vi "testMinMax.vi"(8 "error in (no error)":errorcluster, 10 "passThreshold":i32[](array[numeric]), 11 "reference in":refnum<class "subject.lvclass">) -> (0 "error out":errorcluster, 3 "reference out":refnum<class "subject.lvclass">)   [LabVIEW 2015, in "subject.lvclass"]
uses:
  subject.lvclass
panel:
  in  "valesAmplitude in":dbl[](array[numeric])
  in  "peaksAmplitude in":dbl[](array[numeric])
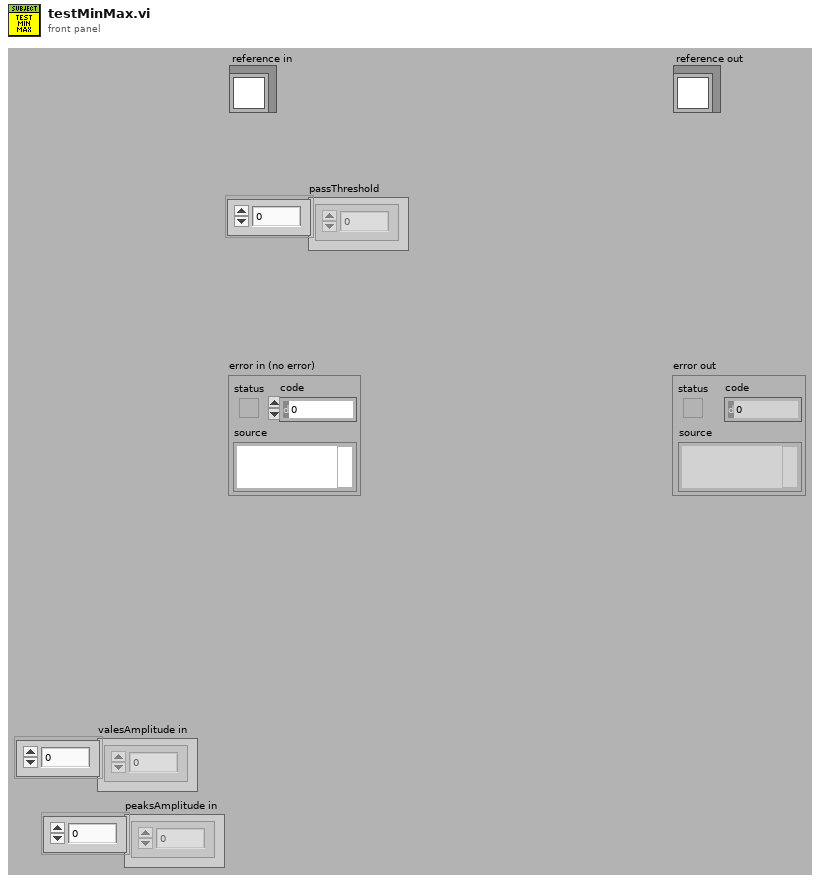
[diagram p1: front panel]
types:
  T1 = cluster{"peaksAmplitude":dbl[], "iPeaksLocation":dbl[], "valesAmplitude":dbl[], "iValesLocation":dbl[], "threshold":dbl, "width_warm":i32, "meanAmpl_warm":i32, "#_peaks":i32}
  T2 = typedef "subject.lvclass/ObjectAttributesRef.ctl" = refnum<data-value>
  T3 = typedef "subject.lvclass/ObjectAttributes.ctl" = cluster{"MyAttribute":dbl, "data":cluster{"Ve_warm":dbl[], "time_warm":dbl[], "name":string, "phase":dbl[], "VCO2":dbl[], "VO2":dbl[], "PetCO2":dbl[], "RQ":dbl[], "HR":dbl[], "Ve_warm_inter":dbl[], "time_warm_inter":dbl[], "Ve_exer":dbl[], "time_exer":dbl[], "Ve_exer_inter":dbl[], "time_exer_inter":dbl[], "Ve":dbl[], "time":dbl[]}, "results_5l":cluster{"EOV":bool, "osci_amplitude":dbl[], "osci_width":dbl[], "peak_location":dbl[], "threshold":dbl, "width":i32}, "results_15percent":cluster{"EOV":bool, "osci_amplitude":dbl[], "osci_width":dbl[], "peak_location":dbl[], "threshold":dbl, "width":i32}, "supportData":cluster{"peaksAmplitude":dbl[], "iPeaksLocation":dbl[], "valesAmplitude":dbl[], "iValesLocation":dbl[], "threshold":dbl, "meanAmpl_warm":i32, "#_peaks":i32, "width":i32}, "results_user_selection":cluster{"EOV":bool, "osci_amplitude":dbl[], "osci_width":dbl[], "peak_location":dbl[], "threshold":dbl, "width":i32}}
  T4 = cluster{"peaksAmplitude":dbl[], "iPeaksLocation":dbl[], "valesAmplitude":dbl[], "iValesLocation":dbl[], "threshold":dbl, "meanAmpl_warm":i32, "#_peaks":i32, "width":i32}
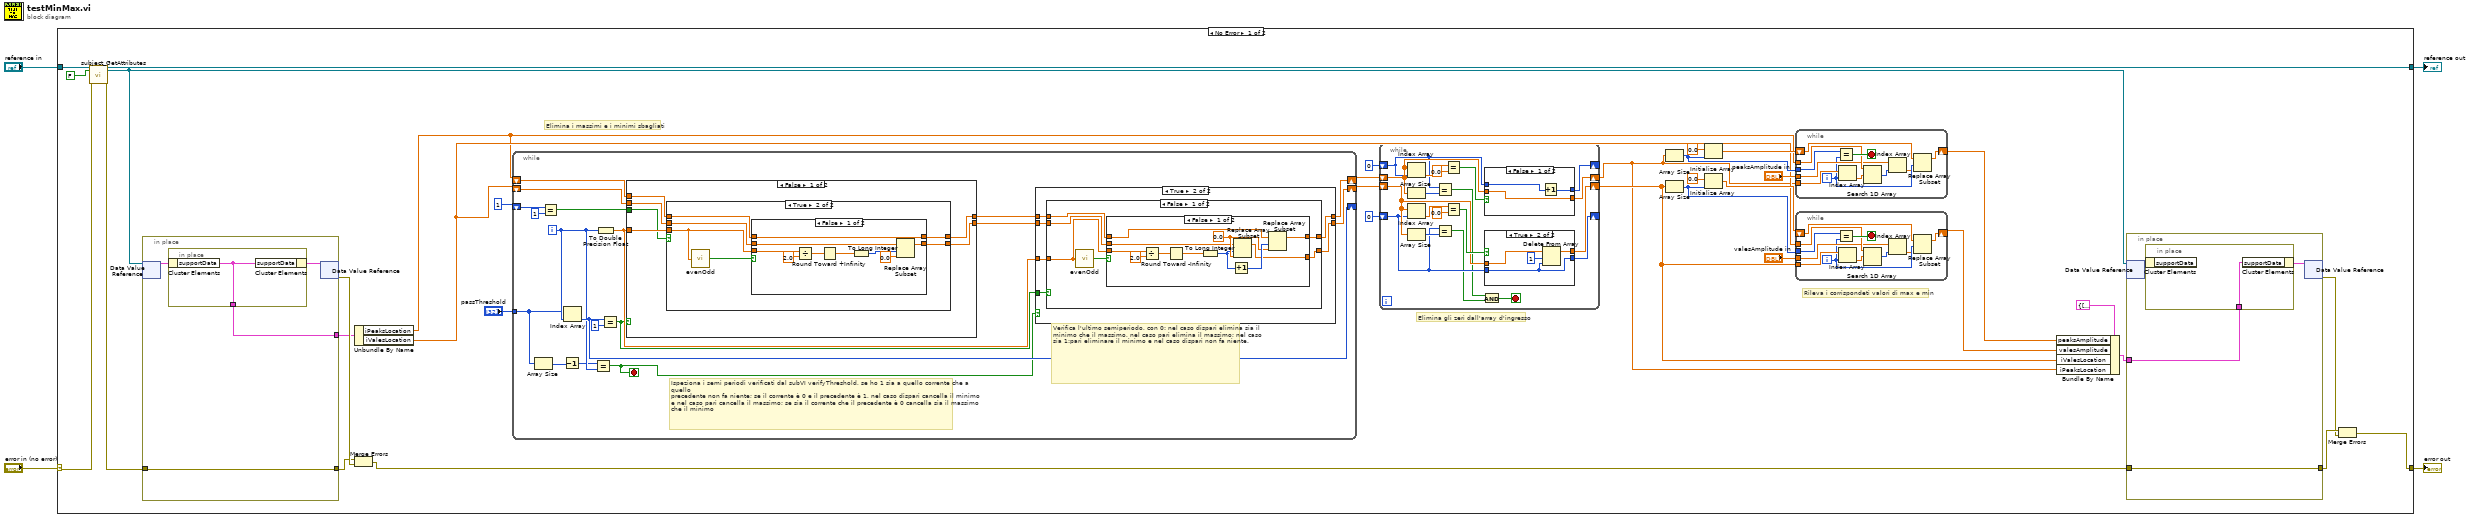
[diagram p0: block diagram]
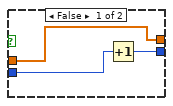
[diagram p2: hidden frame]
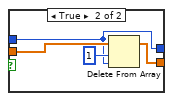
[diagram p3: hidden frame]
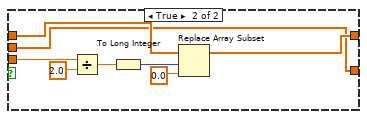
[diagram p5: hidden frame]
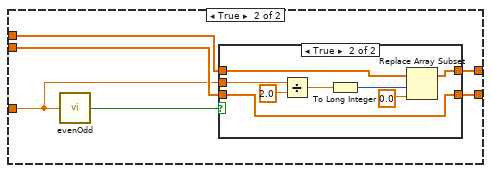
[diagram p6: hidden frame]
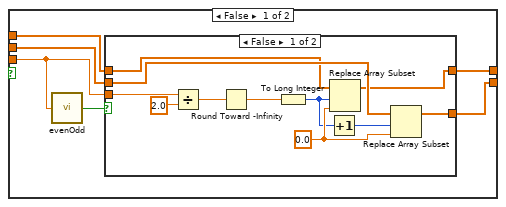
[diagram p8: hidden frame]
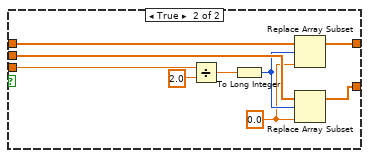
[diagram p9: hidden frame]
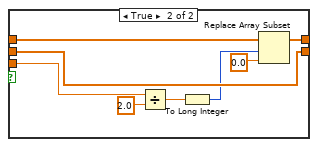
[diagram p10: hidden frame]
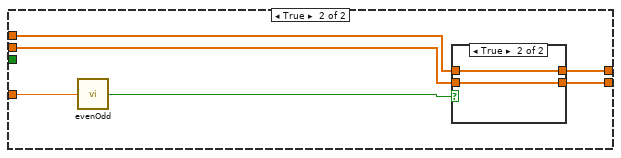
[diagram p11: hidden frame]
diagram:
  n1 = case shown="No Error" "error in (no error)" {
    selector: "error in (no error)" -> [w35 w238]
    tunnel: [w12 w238] -> w3
    tunnel: [w33 w237] -> w1
    tunnel: "reference in" -> [w37 w237]
    frame No Error {
      # "Rileva i corrispondeti valori di max e min"
      # "Elimina gli zeri dall'array d'ingresso"
      # "Elimina i massimi e i minimi sbagliati"
      n2 = call "subject_GetAttributes.vi"("reference in"=w37, "return data? (T)"=FALSE, "error in (no error)"=w35) -> ("reference out"=w33:refnum<class "subject.lvclass">, "attributes ref"=w11:T2, "error out"=w34:errorcluster)  [unwired: 13 in, 1 out]
      n3 = in-place {
        in-place-border: w34 -> [w233]
        in-place-border: [w233] -> w38
        in-place-border: [w232] -> w18
        n4 = in-place-dvr #1(w11) -> (w234:T3)  [unwired: 1 out]
        n5 = in-place {
          in-place-border: [w236] -> w232
          n6 = in-place-cluster #2(w234) -> ("supportData"=w236:T4)
          n7 = in-place-cluster #2("supportData"=w236) -> (w235:T3)
        }
        n8 = in-place-dvr #1(w235) -> (w39:errorcluster)  [unwired: 1 out]
      }
      n9 = Unbundle By Name(w18) -> ("iPeaksLocation"=w16:dbl[], "iValesLocation"=w17:dbl[])
      n10 = Merge Errors(w38, w39) -> (w15:errorcluster)
      n11 = while {
        tunnel: "passThreshold" -> [w101]
        shift-right: [w104] -> w29
        shift-left: w16 -> [w116]
        shift-right: [w105] -> w30
        shift-left: w17 -> [w115]
        shift-right: [w114] -> _
        shift-left: 1 ("element") -> [w113]
        i -> [w110]
        stop <- w106 stop-if-true
        # "Verifica l'ultimo semiperiodo, con 0: nel caso dispari elimina sia il minimo che il massimo, nel caso pari elimina il massimo; nel caso sia 1:pari eliminare il minimo e nel caso dispari non fa niente."
        # "Ispeziona i semi periodi verificati dal subVI verifyThreshold, se ho 1 sia a quello corrente che a quello \nprecedente non fa niente; se il corrente è 0 e il precedente è 1, nel caso dispari cancella il minimo e nel caso pari cancella il massimo; se sia il corrente che il precedente è 0 cancella sia il massimo che il minimo"
        n12 = Array Size(array=w101) -> (size(s)=w109:i32)
        n13 = Equal?(x=w113, y=1) -> (x = y?=w111:bool)
        n14 = Decrement(x=w109) -> (x-1=w103:i32)
        n15 = Index Array(array=w101, index=w110) -> (element=w114:i32)
        n16 = Equal?(x=w103, y=w110) -> (x = y?=w106:bool)
        n17 = To Double Precision Float(number=w110) -> (double precision float=w102:dbl)
        n18 = Equal?(x=w114, y=1) -> (x = y?=w100:bool)
        n19 = case shown="False" w100 {
          tunnel: w102 -> [w172 w227]
          tunnel: w116 -> [w171 w225]
          tunnel: w115 -> [w170 w223]
          tunnel: [w169 w224] -> w107
          tunnel: [w168 w222] -> w108
          tunnel: w111 -> [w167 _]
          frame False {
            n20 = case shown="True" w167 {
              tunnel: w172 -> [w173 w199]
              tunnel: w171 -> [w176 w203]
              tunnel: w170 -> [w178 w200]
              tunnel: [w175 w202] -> w169
              tunnel: [w177 w201] -> w168
              frame False {
                n21 = call "evenOdd.vi"("number"=w173) -> ("odd/even"=w174:bool)
                n22 = case shown="False" w174 {
                  tunnel: w178 -> [w189 w198]
                  tunnel: [w188 w197] -> w177
                  tunnel: w176 -> [w179 w196]
                  tunnel: [w187 w195] -> w175
                  tunnel: w173 -> [w186 w194]
                  frame False {
                    w182 = 0.0 ("new element/subarray")
                    n23 = Divide(x=w186, y=2.0) -> (x/y=w184:dbl)
                    n24 = Round Toward -Infinity(1:w184) -> (0:w183:dbl)
                    n25 = To Long Integer(number=w183) -> (32bit integer=w181:i32)
                    n26 = Increment(x=w181) -> (x+1=w180:i32)
                    n27 = Replace Array Subset(array=w179, new element=w182, index=w181) -> (w187:dbl[])
                    n28 = Replace Array Subset(array=w189, new element=w182, index=w180) -> (w188:dbl[])
                  }
                  frame True {
                    w190 = 0.0 ("new element/subarray")
                    n29 = Divide(x=w194, y=2.0) -> (x/y=w192:dbl)
                    n30 = To Long Integer(number=w192) -> (32bit integer=w191:i32)
                    n31 = Replace Array Subset(array=w196, new element=w190, index=w191) -> (w195:dbl[])
                    n32 = Replace Array Subset(array=w198, new element=w190, index=w191) -> (w197:dbl[])
                  }
                }
              }
              frame True {
                n33 = call "evenOdd.vi"("number"=w199) -> ("odd/even"=w204:bool)
                n34 = case shown="False" w204 {
                  tunnel: w203 -> [w211 w221]
                  tunnel: w200 -> [w213 w219]
                  tunnel: w199 -> [w209 w216]
                  tunnel: [w211 w220] -> w202
                  tunnel: [w212 w219] -> w201
                  frame False {
                    n35 = Divide(x=w209, y=2.0) -> (x/y=w207:dbl)
                    n36 = Round Toward +Infinity(x=w207) -> (ceil(x): smallest int >= x=w206:dbl)
                    n37 = To Long Integer(number=w206) -> (32bit integer=w205:i32)
                    n38 = Replace Array Subset(array=w213, new element=0.0 ("new element/subarray"), index=w205) -> (w212:dbl[])
                  }
                  frame True {
                    n39 = Divide(x=w216, y=2.0) -> (x/y=w214:dbl)
                    n40 = To Long Integer(number=w214) -> (32bit integer=w217:i32)
                    n41 = Replace Array Subset(array=w221, new element=0.0 ("length"), index=w217) -> (w220:dbl[])
                  }
                }
              }
            }
          }
          frame True {
            n42 = call "evenOdd.vi"("number"=w227) -> ("odd/even"=w226:bool)
            n43 = case shown="True" w226 {
              tunnel: w225 -> [w229 w231]
              tunnel: [w229 w231] -> w224
              tunnel: w223 -> [w228 w230]
              tunnel: [w228 w230] -> w222
              frame False {
              }
              frame True {
              }
            }
          }
        }
        n44 = case shown="True" w106 {
          tunnel: w108 -> [w119 w125]
          tunnel: w107 -> [w118 w122]
          tunnel: w102 -> [_ w124]
          tunnel: [w119 w123] -> w105
          tunnel: [w118 w121] -> w104
          tunnel: w100 -> [_ w120]
          frame False {
          }
          frame True {
            n45 = case shown="False" w120 {
              tunnel: w125 -> [w130 w155]
              tunnel: w124 -> [w126 w154]
              tunnel: [w128 w153] -> w123
              tunnel: w122 -> [w129 w152]
              tunnel: [w127 w151] -> w121
              frame False {
                n46 = call "evenOdd.vi"("number"=w126) -> ("odd/even"=w131:bool)
                n47 = case shown="False" w131 {
                  tunnel: w130 -> [w136 w148]
                  tunnel: w129 -> [w135 w150]
                  tunnel: [w134 w148] -> w128
                  tunnel: [w133 w149] -> w127
                  tunnel: w126 -> [w132 w147]
                  frame False {
                    w141 = 0.0 ("new element/subarray")
                    n48 = Divide(x=w132, y=2.0) -> (x/y=w138:dbl)
                    n49 = Round Toward -Infinity(1:w138) -> (0:w139:dbl)
                    n50 = To Long Integer(number=w139) -> (32bit integer=w140:i32)
                    n51 = Increment(x=w140) -> (x+1=w142:i32)
                    n52 = Replace Array Subset(array=w136, new element=w141, index=w140) -> (w134:dbl[])
                    n53 = Replace Array Subset(array=w135, new element=w141, index=w142) -> (w133:dbl[])
                  }
                  frame True {
                    n54 = Divide(x=w147, y=2.0) -> (x/y=w145:dbl)
                    n55 = To Long Integer(number=w145) -> (32bit integer=w144:i32)
                    n56 = Replace Array Subset(array=w150, new element=0.0 ("new element/subarray"), index=w144) -> (w149:dbl[])
                  }
                }
              }
              frame True {
                n57 = call "evenOdd.vi"("number"=w154) -> ("odd/even"=w156:bool)
                n58 = case shown="True" w156 {
                  tunnel: w155 -> [w157 w159]
                  tunnel: w154 -> [_ w166]
                  tunnel: [w157 w159] -> w153
                  tunnel: w152 -> [w158 w161]
                  tunnel: [w158 w160] -> w151
                  frame False {
                  }
                  frame True {
                    n59 = Divide(x=w166, y=2.0) -> (x/y=w164:dbl)
                    n60 = To Long Integer(number=w164) -> (32bit integer=w163:i32)
                    n61 = Replace Array Subset(array=w161, new element=0.0 ("new element/subarray"), index=w163) -> (w160:dbl[])
                  }
                }
              }
            }
          }
        }
      }
      n62 = while {
        shift-right: [w78] -> w7
        shift-left: w29 -> [w71]
        shift-right: [w79] -> w8
        shift-left: w30 -> [w75]
        shift-right: [w77] -> _
        shift-left: 0 -> [w73]
        shift-right: [w76] -> _
        shift-left: 0 -> [w67]
        stop <- w68 stop-if-true
        n63 = Index Array(array=w71, index=w67) -> (element=w85:dbl)
        n64 = Array Size(array=w71) -> (size(s)=w72:i32)
        n65 = Index Array(array=w75, index=w73) -> (element=w82:dbl)
        n66 = Array Size(array=w75) -> (size(s)=w74:i32)
        n67 = Equal?(x=w67, y=w72) -> (x = y?=w69:bool)
        n68 = Equal?(x=w73, y=w74) -> (x = y?=w70:bool)
        n69 = Equal?(x=w85, y=0.0) -> (x = y?=w83:bool)
        n70 = Equal?(x=w82, y=0.0) -> (x = y?=w80:bool)
        n71 = And(x=w69, y=w70) -> (x .and. y?=w68:bool)
        n72 = case shown="False" w83 {
          tunnel: w71 -> [w93 w99]
          tunnel: [w93 w98] -> w78
          tunnel: [w95 w96] -> w76
          tunnel: w67 -> [w94 w96]
          frame False {
            n73 = Increment(x=w94) -> (x+1=w95:i32)
          }
          frame True {
            n74 = Delete From Array(array=w99, length=1, index=w96) -> (array with subset deleted=w98:dbl[])  [unwired: 1 out]
          }
        }
        n75 = case shown="True" w80 {
          tunnel: w75 -> [w86 w92]
          tunnel: [w86 w91] -> w79
          tunnel: [w88 w89] -> w77
          tunnel: w73 -> [w87 w89]
          frame False {
            n76 = Increment(x=w87) -> (x+1=w88:i32)
          }
          frame True {
            n77 = Delete From Array(array=w92, length=1, index=w89) -> (array with subset deleted=w91:dbl[])  [unwired: 1 out]
          }
        }
      }
      n78 = Array Size(array=w7) -> (size(s)=w25:i32)
      n79 = Array Size(array=w8) -> (size(s)=w22:i32)
      n80 = Initialize Array(0.0 ("element"), w25) -> (w23:dbl[])
      n81 = Initialize Array(0.0 ("element"), w22) -> (w20:dbl[])
      n82 = while {
        tunnel: w16 -> [w63]
        tunnel: w7 -> [w65]
        tunnel: "peaksAmplitude in" -> [w61]
        tunnel: w25 -> [w62]
        shift-right: [w58] -> w6
        shift-left: w23 -> [w59]
        i -> [w57]
        stop <- w66 stop-if-true
        n83 = Equal?(x=w62, y=w57) -> (x = y?=w66:bool)
        n84 = Index Array(array=w65, index=w57) -> (element=w64:dbl)
        n85 = Search 1D Array(1D array=w63, element=w64) -> (index of element=w60:i32)  [unwired: 1 in]
        n86 = Index Array(array=w61, index=w60) -> (element=w56:dbl)
        n87 = Replace Array Subset(array=w59, new element=w56, index=w57) -> (w58:dbl[])
      }
      n88 = while {
        tunnel: w17 -> [w52]
        tunnel: w8 -> [w54]
        tunnel: "valesAmplitude in" -> [w50]
        tunnel: w22 -> [w51]
        shift-right: [w47] -> w5
        shift-left: w20 -> [w48]
        i -> [w46]
        stop <- w55 stop-if-true
        n89 = Equal?(x=w51, y=w46) -> (x = y?=w55:bool)
        n90 = Index Array(array=w54, index=w46) -> (element=w53:dbl)
        n91 = Search 1D Array(1D array=w52, element=w53) -> (index of element=w49:i32)  [unwired: 1 in]
        n92 = Index Array(array=w50, index=w49) -> (element=w45:dbl)
        n93 = Replace Array Subset(array=w48, new element=w45, index=w46) -> (w47:dbl[])
      }
      n94 = Bundle By Name(cluster=T1 {"peaksAmplitude"=[], "iPeaksLocation"=[], "valesAmplitude"=[], "iValesLocation"=[], "threshold"=0.0, "width_warm"=0, "meanAmpl_warm"=0, "#_peaks"=0} ("supportData"), "peaksAmplitude"=w6, "valesAmplitude"=w5, "iValesLocation"=w8, "iPeaksLocation"=w7) -> (w9:T1)
      n95 = in-place {
        in-place-border: w15 -> [w41]
        in-place-border: [w41] -> w14
        in-place-border: w9 -> [w40]
        n96 = in-place-dvr #3(w11) -> (w42:T3)  [unwired: 1 out]
        n97 = in-place {
          in-place-border: w40 -> [w44]
          n98 = in-place-cluster #4(w42) -> ()  [unwired: 1 out]
          n99 = in-place-cluster #4("supportData"=w44) -> (w43:T3)
        }
        n100 = in-place-dvr #3(w43) -> (w13:errorcluster)  [unwired: 1 out]
      }
      n101 = Merge Errors(w14, w13) -> (w12:errorcluster)
    }
    frame Error {
    }
  }
  "error out" <- w3
  "reference out" <- w1
